vi "Set Slit Width.vi"(8 "error in (no error)":errorcluster, 10 "Slit Width (um)":i32, 11 "VISA resource name":refnum<visa-resource-name>) -> (0 "error out":errorcluster, 3 "VISA resource name out":refnum<visa-resource-name>, 4 "read buffer":string)   [LabVIEW 2019, in "SpectraPro.lvlib"]
uses:
  SpectraPro.lvlib
panel:
  out "output":string
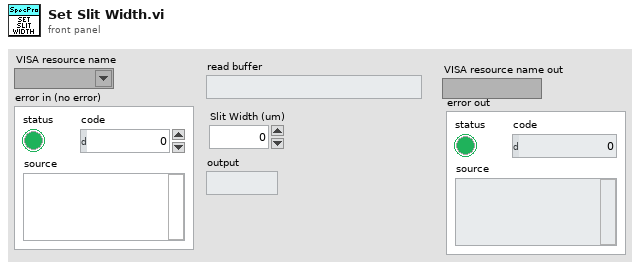
[diagram p1: front panel]
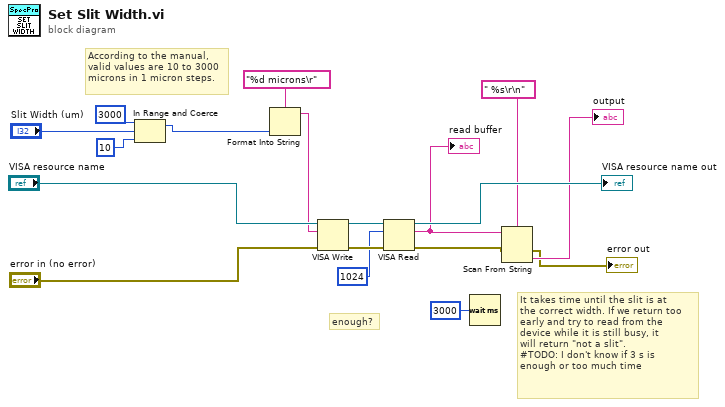
[diagram p0: block diagram]
diagram:
  # "It takes time until the slit is at\nthe correct width. If we return too\nearly and try to read from the\ndevice while it is still busy, it\nwill return \"not a slit\".\n#TODO: I don't know if 3 s is\nenough or too much time"
  # "According to the manual,\nvalid values are 10 to 3000\nmicrons in 1 micron steps."
  # "enough?"
  n1 = In Range and Coerce(upper limit=3000, x="Slit Width (um)", lower limit=10) -> (coerced(x)=w6:i32)  [unwired: 1 out]
  n2 = Format Into String(format string="%d microns\r" ("write buffer"), w6) -> (resulting string=w8:string)  [unwired: 2 in, 1 out]
  n3 = VISA Write(VISA resource name="VISA resource name", write buffer=w8, error in (no error)="error in (no error)") -> (VISA resource name out=w16:refnum<visa-resource-name>, error out=w17:errorcluster)  [unwired: 1 out]
  n4 = VISA Read(VISA resource name=w16, byte count=u32 1024, error in (no error)=w17) -> (VISA resource name out=→"VISA resource name out":refnum<visa-resource-name>, read buffer=w12:string, error out=w3:errorcluster)  [unwired: 1 out]
  "read buffer" <- w12
  n5 = Wait (ms)(milliseconds to wait=u32 3000) -> ()  [unwired: 1 out]
  n6 = Scan From String(format string=" %s\r\n", input string=w12, error in=w3) -> (error out=→"error out":errorcluster, output 1=→"output":string)  [unwired: 2 in, 2 out]
